vi "Laser-Get-Shotstatus.vi"(0 "VISA resource name":refnum<visa-resource-name>, 1 "error in (no error)":errorcluster) -> (2 "VISA resource name out":refnum<visa-resource-name>, 3 "cluster":T1, 4 "error out":errorcluster)   [LabVIEW 2013]
panel:
  out "array w/ subset deleted":bool[](array[boolean])
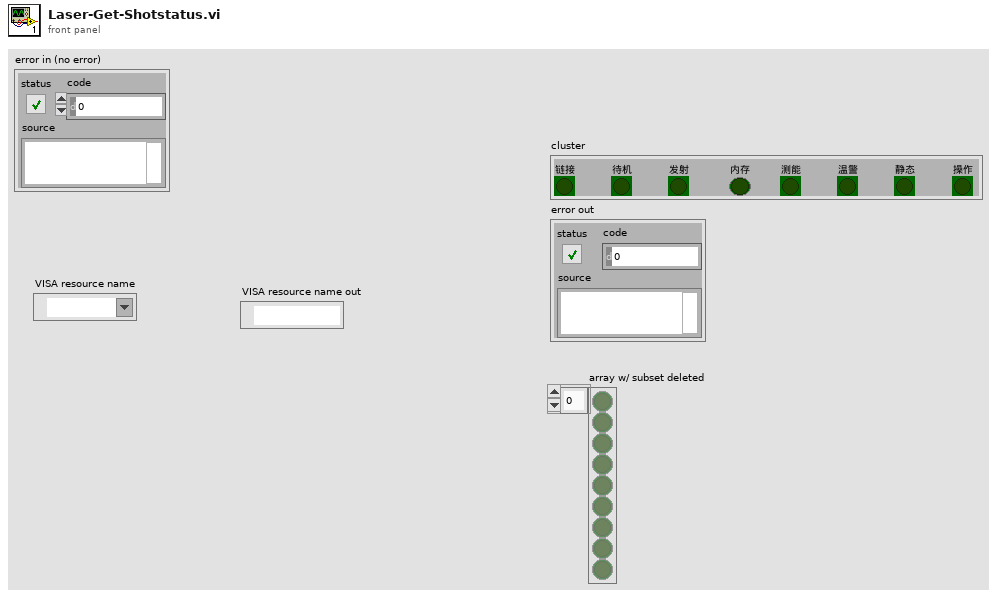
[diagram p1: front panel]
types:
  T1 = cluster{"链接":bool, "待机":bool, "发射":bool, "[3]":bool, "内存":bool, "测能":bool, "温警":bool, "静态":bool, "操作":bool}
  T2 = cluster{"[0]":bool, "[1]":bool, "[2]":bool, "[3]":bool, "[4]":bool, "[5]":bool, "[6]":bool, "[7]":bool, "[8]":bool}
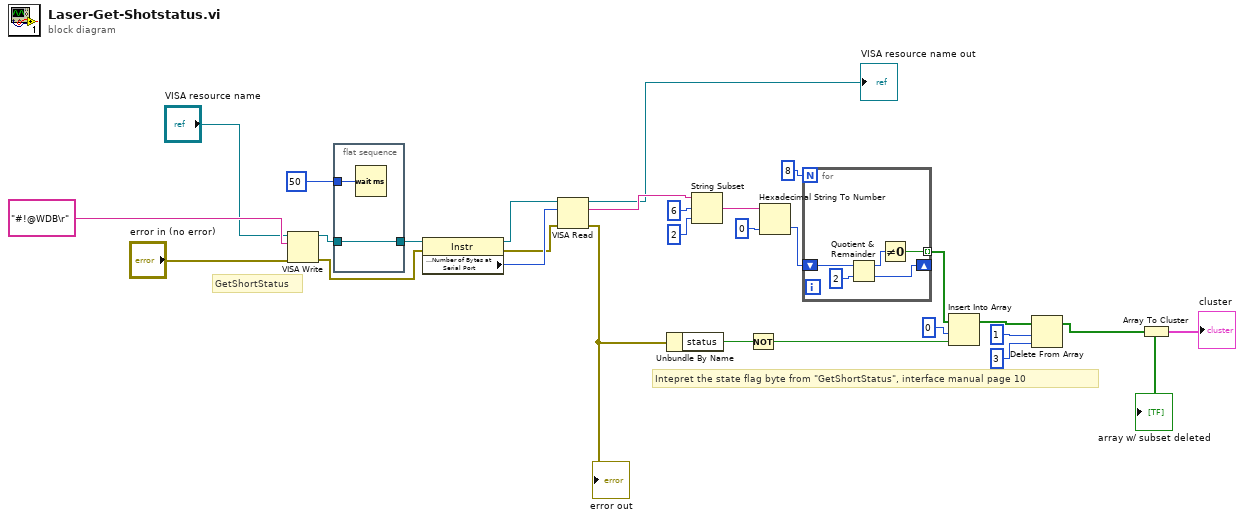
[diagram p0: block diagram]
diagram:
  # "Intepret the state flag byte from \"GetShortStatus\", interface manual page 10"
  # "GetShortStatus"
  n1 = VISA Write(VISA resource name="VISA resource name", write buffer="#!@WDB\r", error in (no error)="error in (no error)") -> (VISA resource name out=w23:refnum<visa-resource-name>, error out=w3:errorcluster)  [unwired: 1 out]
  n2 = flat-sequence {
    tunnel: w23 -> [w29]
    tunnel: [w29] -> w24
    tunnel: u32 50 ("delay before read (ms)") -> [w30]
    frame #0 {
      n3 = Wait (ms)(milliseconds to wait=w30) -> ()  [unwired: 1 out]
    }
  }
  n4 = property class="Instr"(reference=w24, error in=w3) -> (reference out=w25:refnum<visa-resource-name>, error out=w26:errorcluster, "Serial Settings:Number of Bytes at Serial Port"=w27:u32)
  n5 = VISA Read(VISA resource name=w25, byte count=w27, error in (no error)=w26) -> (VISA resource name out=→"VISA resource name out":refnum<visa-resource-name>, read buffer=w21:string, error out=w2:errorcluster)  [unwired: 1 out]
  "error out" <- w2
  n6 = Unbundle By Name(w2) -> ("status"=w17:bool)
  n7 = String Subset(string=w21, offset (0)=6, length (rest)=2 ("length (rest)")) -> (substring=w10:string)
  n8 = Not(x=w17) -> (.not. x?=w16:bool)
  n9 = Hexadecimal String To Number(string=w10, default (0uL)=u8 0 ("default (0 U32)")) -> (number=w11:u8)  [unwired: 1 in, 1 out]
  n10 = for {
    N: 8 -> [_]
    tunnel: [w33] -> w8 mode=indexing
    shift-right: [w32] -> _
    shift-left: w11 -> [w31]
    n11 = Quotient & Remainder(x=w31, y=2) -> (x-y*floor(x/y)=w34:i32, floor(x/y)=w32:i32)
    n12 = Not Equal To 0?(x=w34) -> (x != 0?=w33:bool)
  }
  n13 = Insert Into Array "Insert Into Array"(array=w8, index=0, new element=w16) -> (w9:bool[])
  n14 = Delete From Array "Delete From Array"(array=w9, length=1, index=3) -> (array with subset deleted=w5:bool[])  [unwired: 1 out]
  "array w/ subset deleted" <- w5
  n15 = Array To Cluster(array=w5) -> (cluster=→"cluster":T2)
